vi "Update Object.vi"(8 "error in (no error)":errorcluster, 10 "SerializableObject in":refnum<class "SerializableObject.lvclass">, 11 "Editor.lvclass in":refnum<data-value>) -> (0 "error out":errorcluster, 3 "Editor.lvclass out":refnum<data-value>)   [LabVIEW 2015, in "Editor.lvclass"]
uses:
  Editor.lvclass
  SerializableObject/SerializableObject.lvclass
  Project.lvclass
  Step.lvclass
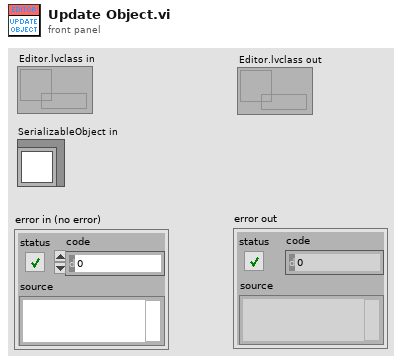
[diagram p1: front panel]
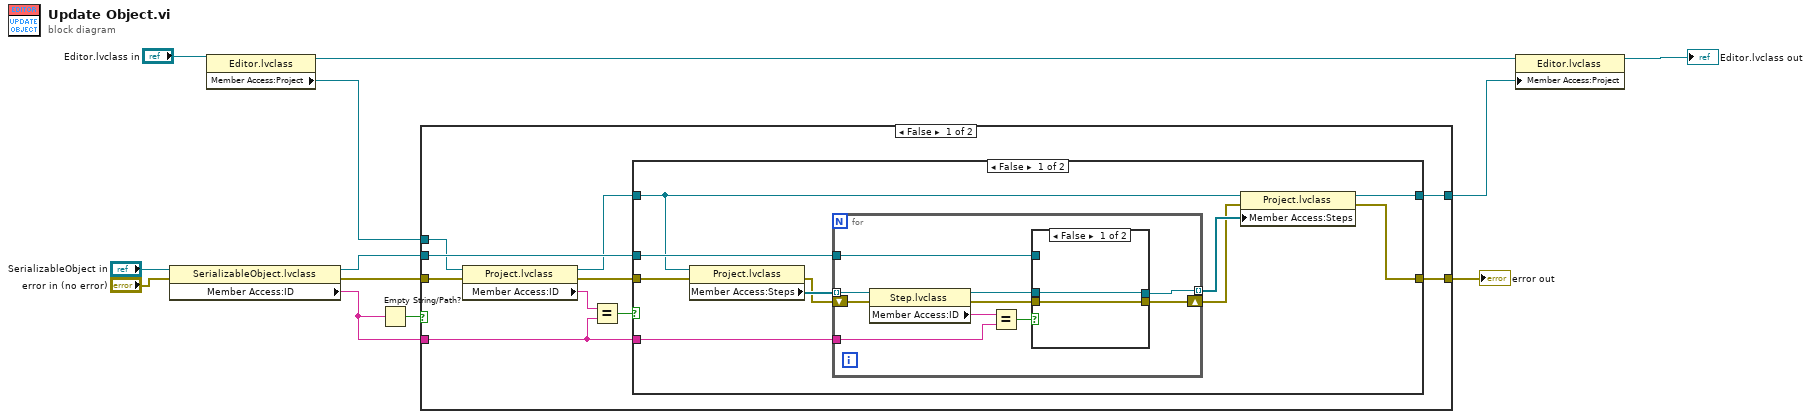
[diagram p0: block diagram]
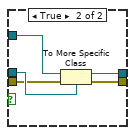
[diagram p2: hidden frame]
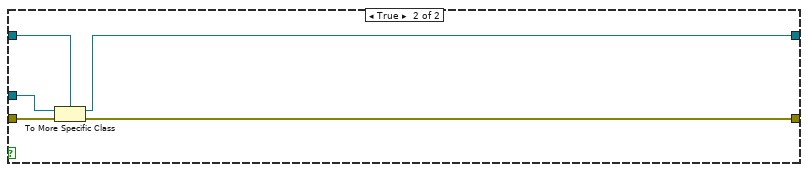
[diagram p3: hidden frame]
diagram:
  n1 = property class="SerializableObject.lvclass"(reference="SerializableObject in", error in="error in (no error)") -> (reference out=w7:refnum<class "SerializableObject.lvclass">, error out=w9:errorcluster, "Member Access:ID"=w8:string)
  n2 = property class="Editor.lvclass"(reference="Editor.lvclass in") -> (reference out=w3:refnum<data-value>, "Member Access:Project"=w4:refnum<class "Project.lvclass">)  [unwired: 1 in, 1 out]
  n3 = Empty String/Path?(string/path=w8) -> (empty?=w10:bool)
  n4 = case shown="False" w10 {
    tunnel: w9 -> [w22 w55]
    tunnel: w4 -> [w15 w56]
    tunnel: w8 -> [w16 _]
    tunnel: w7 -> [w19 _]
    tunnel: [w14 w56] -> w2
    tunnel: [w13 w55] -> w6
    frame False {
      n5 = property class="Project.lvclass"(reference=w15, error in=w22) -> (reference out=w18:refnum<class "Project.lvclass">, error out=w17:errorcluster, "Member Access:ID"=w21:string)
      n6 = Equal?(x=w21, y=w16) -> (x = y?=w20:bool)
      n7 = case shown="False" w20 {
        tunnel: w19 -> [w28 w53]
        tunnel: w18 -> [w27 w52]
        tunnel: w17 -> [w32 w54]
        tunnel: w16 -> [w31 _]
        tunnel: [w24 w51] -> w13
        tunnel: [w23 w50] -> w14
        frame False {
          n8 = property class="Project.lvclass"(reference=w27, error in=w32) -> (error out=w29:errorcluster, "Member Access:Steps"=w30:refnum<class "Step.lvclass">[])  [unwired: 1 out]
          n9 = for {
            tunnel: w31 -> [w39]
            tunnel: w30 -> [w42] mode=indexing
            tunnel: w28 -> [w35]
            tunnel: [w34] -> w26 mode=indexing
            shift-right: [w33] -> w25
            shift-left: w29 -> [w40]
            n10 = property class="Step.lvclass"(reference=w42, error in=w40) -> (reference out=w36:refnum<class "Step.lvclass">, error out=w37:errorcluster, "Member Access:ID"=w41:string)
            n11 = Equal?(x=w41, y=w39) -> (x = y?=w38:bool)
            n12 = case shown="False" w38 {
              tunnel: w37 -> [w43 w47]
              tunnel: w36 -> [w44 w48]
              tunnel: w35 -> [_ w49]
              tunnel: [w44 w46] -> w34
              tunnel: [w43 w45] -> w33
              frame False {
              }
              frame True {
                n13 = To More Specific Class(target class=w48, reference=w49, error in=w47) -> (specific class reference=w46:refnum<class "Step.lvclass">, error out=w45:errorcluster)
              }
            }
          }
          n14 = property class="Project.lvclass"(reference=w27, error in=w25, "Member Access:Steps"=w26) -> (reference out=w23:refnum<class "Project.lvclass">, error out=w24:errorcluster)
        }
        frame True {
          n15 = To More Specific Class(target class=w52, reference=w53, error in=w54) -> (specific class reference=w50:refnum<class "Project.lvclass">, error out=w51:errorcluster)
        }
      }
    }
    frame True {
    }
  }
  "error out" <- w6
  n16 = property class="Editor.lvclass"(reference=w3, "Member Access:Project"=w2) -> (reference out=→"Editor.lvclass out":refnum<data-value>)  [unwired: 1 in, 1 out]
